vi "20211022_HW01.vi"() -> ()   [LabVIEW 2019]
panel:
  out "T":i32
  in  "N":i32
  # "N=0~100, T=N+10\nN=-50~1, T=abs(N)\nN>100, T=T^2\nN<-50, T=T-N"
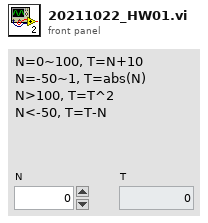
[diagram p1: front panel]
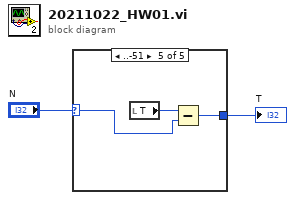
[diagram p0: block diagram]
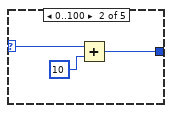
[diagram p3: hidden frame]
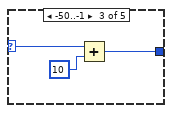
[diagram p4: hidden frame]
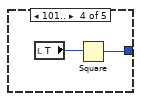
[diagram p5: hidden frame]
diagram:
  n1 = case shown="..-51" "N" {
    selector: "N" -> [w3 w6 w9 _ w12]
    tunnel: [w3 w4 w7 w10 w13] -> w1
    frame Default {
    }
    frame 0..100 {
      n2 = Add(x=w6, y=10) -> (x+y=w4:i32)
    }
    frame -50..-1 {
      n3 = Add(x=w9, y=10) -> (x+y=w7:i32)
    }
    frame 101.. {
      n4 = local read "T"() -> (w11:i32)
      n5 = Square(x=w11) -> (x^2=w10:i32)
    }
    frame ..-51 {
      n6 = local read "T"() -> (w14:i32)
      n7 = Subtract(x=w14, y=w12) -> (x-y=w13:i32)
    }
  }
  "T" <- w1
